vi "test_struc.vi"() -> ()   [LabVIEW 2021]
uses:
  dependencies_dll_release/TCV_Lib.dll
panel:
  out "Cluster":T1
  out "numDet 2":i32
  out "success":i32
  in  "model_h":i32=736
  in  "device":u64=1
  in  "iou":dbl=0.6
  in  "conf":dbl=0.4
  in  "frame_w":u64=1280
  in  "frame_h":u64=736
  in  "model_w":u64=1280
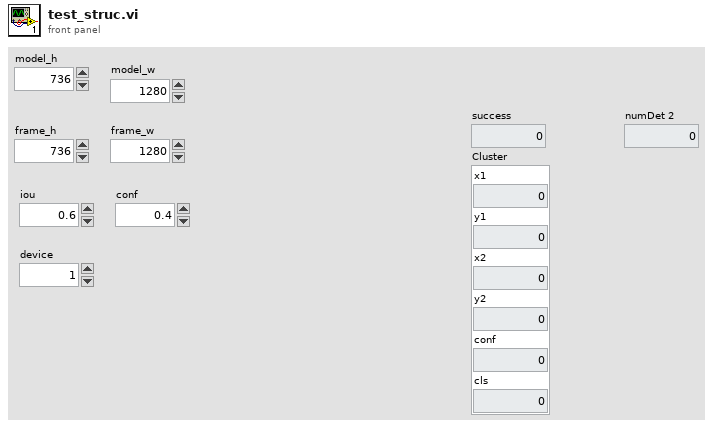
[diagram p1: front panel]
types:
  T1 = cluster{"x1":sgl, "y1":sgl, "x2":sgl, "y2":sgl, "conf":sgl, "cls":i32}
  T2 = cluster{"x1":sgl, "y1":sgl, "x2":sgl, "y2":sgl, "conf":sgl, "cls":i32}[]
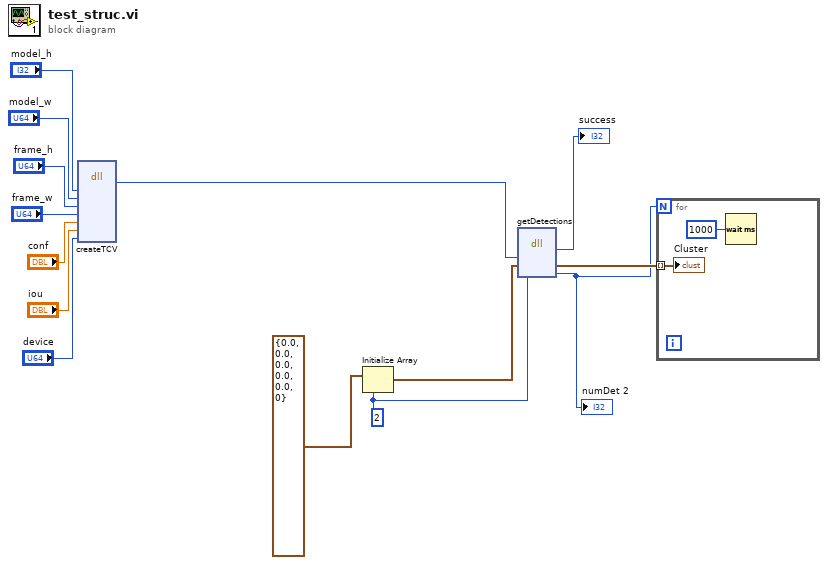
[diagram p0: block diagram]
diagram:
  w1 = 2 ("dimension size")
  n1 = dll-call lib="D:/labviewTestTCVdll/TransformCV-LabVIEW/Test/dependencies_dll_release/TCV_Lib.dll" fn="createTCV"("m_h"="model_h", "m_w"="model_w", "f_h"="frame_h", "f_w"="frame_w", "conf"="conf", "iou"="iou", "device"="device") -> ("returnObj"=w6:u64)  [unwired: 10 in, 2 out]
  n2 = Initialize Array(T1 {"x1"=0.0, "y1"=0.0, "x2"=0.0, "y2"=0.0, "conf"=0.0, "cls"=0}, w1) -> (w5:T2)
  n3 = dll-call lib="D:/labviewTestTCVdll/TransformCV-LabVIEW/Test/dependencies_dll_release/TCV_Lib.dll" fn="getDetections"("ref"=w6, "cluster"=w5, "numDet"=w1) -> ("success"=→"success":i32, "cluster"=w3:T2, "numDet"=w2:i32)  [unwired: 4 in, 2 out]
  "numDet 2" <- w2
  n4 = for {
    N: w2 -> [_]
    tunnel: w3 -> [w16] mode=indexing
    n5 = Wait (ms)(milliseconds to wait=u32 1000) -> ()  [unwired: 1 out]
    "Cluster" <- w16
  }
